vi "Cleanup.vi"(8 "error in":errorcluster, 11 "WAMP Client in":refnum<class "WAMP Client.lvclass">) -> (0 "error out":errorcluster, 3 "WAMP Client out":refnum<class "WAMP Client.lvclass">)   [LabVIEW 2020, in "wamplv.lvlib" / "WAMP Client.lvclass"]
uses:
  WAMP Client.lvclass
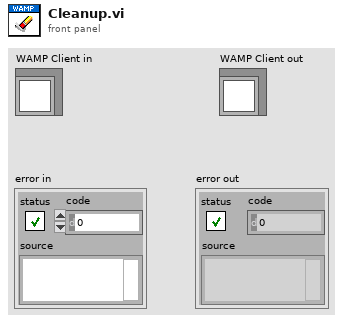
[diagram p1: front panel]
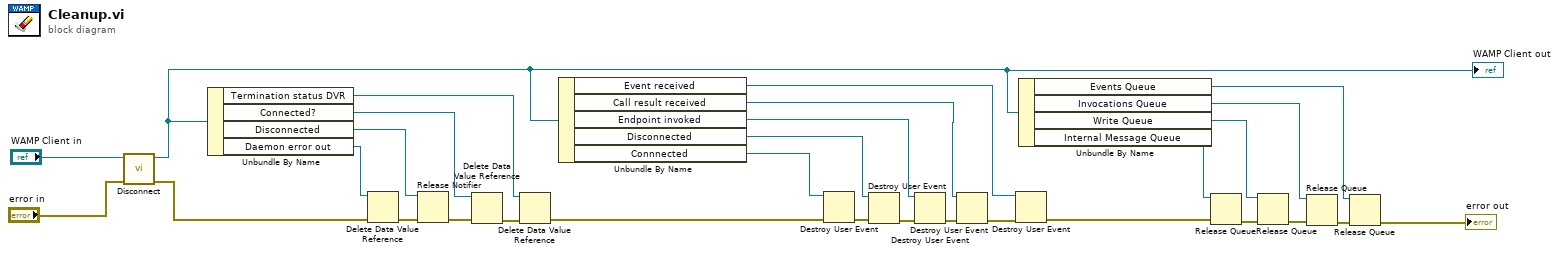
[diagram p0: block diagram]
diagram:
  n1 = call-dynamic "Disconnect.vi"("error in"="error in", "WAMP Client in"="WAMP Client in") -> ("error out"=w2:errorcluster, "WAMP Client out"=w19:refnum<class "WAMP Client.lvclass">)  [unwired: 8 in]
  "WAMP Client out" <- w19
  n2 = Unbundle By Name(w19) -> ("Termination status DVR"=w27:refnum<data-value>, "Connected?"=w30:refnum<data-value>, "Disconnected"=w25:refnum<notifier>, "Daemon error out"=w3:refnum<data-value>)
  n3 = Delete Data Value Reference(data value reference=w3, error in=w2) -> (error out=w1:errorcluster)  [unwired: 1 out]
  n4 = Release Notifier(notifier=w25, error in (no error)=w1) -> (error out=w26:errorcluster)  [unwired: 1 in, 2 out]
  n5 = Delete Data Value Reference(data value reference=w30, error in=w26) -> (error out=w28:errorcluster)  [unwired: 1 out]
  n6 = Delete Data Value Reference(data value reference=w27, error in=w28) -> (error out=w5:errorcluster)  [unwired: 1 out]
  n7 = Unbundle By Name(w19) -> ("Event received"=w14:refnum<user-event>, "Call result received"=w15:refnum<user-event>, "Endpoint invoked"=w16:refnum<user-event>, "Disconnected"=w7:refnum<user-event>, "Connnected"=w6:refnum<user-event>)
  n8 = Destroy User Event(user event=w6, error in=w5) -> (error out=w8:errorcluster)
  n9 = Destroy User Event(user event=w7, error in=w8) -> (error out=w9:errorcluster)
  n10 = Destroy User Event(user event=w16, error in=w9) -> (error out=w18:errorcluster)
  n11 = Destroy User Event(user event=w15, error in=w18) -> (error out=w17:errorcluster)
  n12 = Destroy User Event(user event=w14, error in=w17) -> (error out=w4:errorcluster)
  n13 = Unbundle By Name(w19) -> ("Events Queue"=w21:refnum<queue>, "Invocations Queue"=w23:refnum<queue>, "Write Queue"=w10:refnum<queue>, "Internal Message Queue"=w11:refnum<queue>)
  n14 = Release Queue(queue=w11, error in (no error)=w4) -> (error out=w12:errorcluster)  [unwired: 1 in, 2 out]
  n15 = Release Queue(queue=w10, error in (no error)=w12) -> (error out=w13:errorcluster)  [unwired: 1 in, 2 out]
  n16 = Release Queue(queue=w23, error in (no error)=w13) -> (error out=w22:errorcluster)  [unwired: 1 in, 2 out]
  n17 = Release Queue(queue=w21, error in (no error)=w22) -> (error out=→"error out":errorcluster)  [unwired: 1 in, 2 out]
